vi "ObtieneIndexBotones123.vi"(8 "error in (no error)":errorcluster, 10 "Botones":string[](array[string])=["1_D2", "2_D2", "3_D2"], 11 "Prueba21_1 in":refnum<class "Prueba21.lvclass">) -> (0 "error out":errorcluster, 1 "index of element":i32, 3 "Prueba21_1 out":refnum<class "Prueba21.lvclass">)   [LabVIEW 2019, in "Prueba21.lvclass"]
uses:
  Prueba21.lvclass
  Prueba21.lvclass/Prueba21.ctl
  RerenceAllControlsToolkit/_get mutiple control reference by name.vi
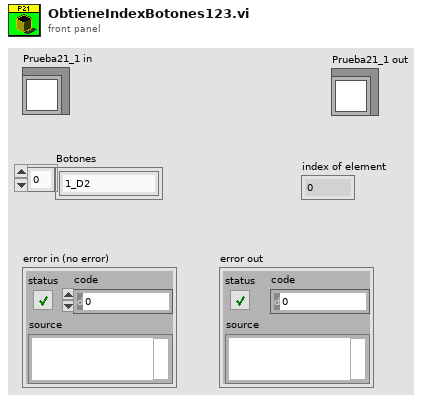
[diagram p1: front panel]
types:
  T1 = cluster{"ControlName":string, "ControlReference":refnum<vi>}[]
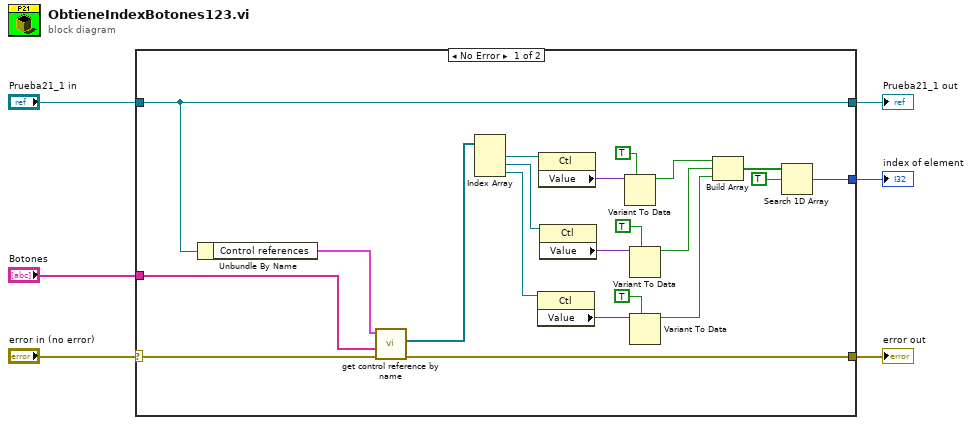
[diagram p0: block diagram]
diagram:
  n1 = case shown="No Error" "error in (no error)" {
    selector: "error in (no error)" -> [w9 w28]
    tunnel: [w14 w28] -> w6
    tunnel: "Prueba21_1 in" -> [w8 w29]
    tunnel: [w10 _] -> w4
    tunnel: [w8 w29] -> w2
    tunnel: "Botones" -> [w7 _]
    frame No Error {
      n2 = Unbundle By Name(w8) -> ("Control references"=w12:T1)
      n3 = call-poly "get control reference by name.vi"("error in (no error)"=w9, "Control names"=w7, "Control references"=w12) -> ("error out"=w14:errorcluster, "References"=w13:refnum<vi>[])  [unwired: 3 in]
      n4 = Index Array(array=w13) -> (element #1=w16:refnum<vi>, element #2=w17:refnum<vi>, element #3=w18:refnum<vi>)  [unwired: 3 in]
      n5 = property class="Ctl"(reference=w18) -> ("Value"=w21:variant)  [unwired: 1 in, 2 out]
      n6 = property class="Ctl"(reference=w16) -> ("Value"=w19:variant)  [unwired: 1 in, 2 out]
      n7 = property class="Ctl"(reference=w17) -> ("Value"=w20:variant)  [unwired: 1 in, 2 out]
      n8 = Variant To Data(type=TRUE, Variant=w19) -> (data=w25:bool)  [unwired: 1 in, 1 out]
      n9 = Variant To Data(type=TRUE, Variant=w20) -> (data=w26:bool)  [unwired: 1 in, 1 out]
      n10 = Variant To Data(type=TRUE, Variant=w21) -> (data=w27:bool)  [unwired: 1 in, 1 out]
      n11 = Build Array(w25, w26, w27) -> (w11:bool[])
      n12 = Search 1D Array(1D array=w11, element=TRUE) -> (index of element=w10:i32)  [unwired: 1 in]
    }
    frame Error {
    }
  }
  "error out" <- w6
  "index of element" <- w4
  "Prueba21_1 out" <- w2
